vi "Update p PAA25.vi"(8 "error in":errorcluster, 10 "p PAA-25":waveform(dbl)[](array[waveform]), 11 "DeepU Results in":refnum<class "DeepU Results.lvclass">) -> (0 "error out":errorcluster, 3 "DeepU Results out":refnum<class "DeepU Results.lvclass">)   [LabVIEW 2019, in "Results.lvlib" / "DeepU Results.lvclass"]
uses:
  DeepU Results.lvclass
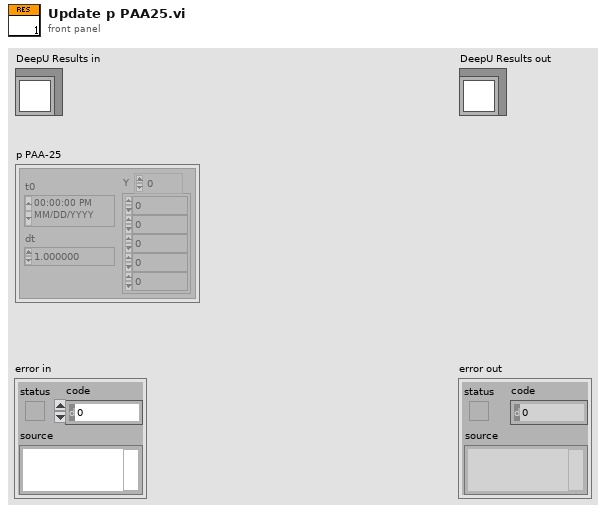
[diagram p1: front panel]
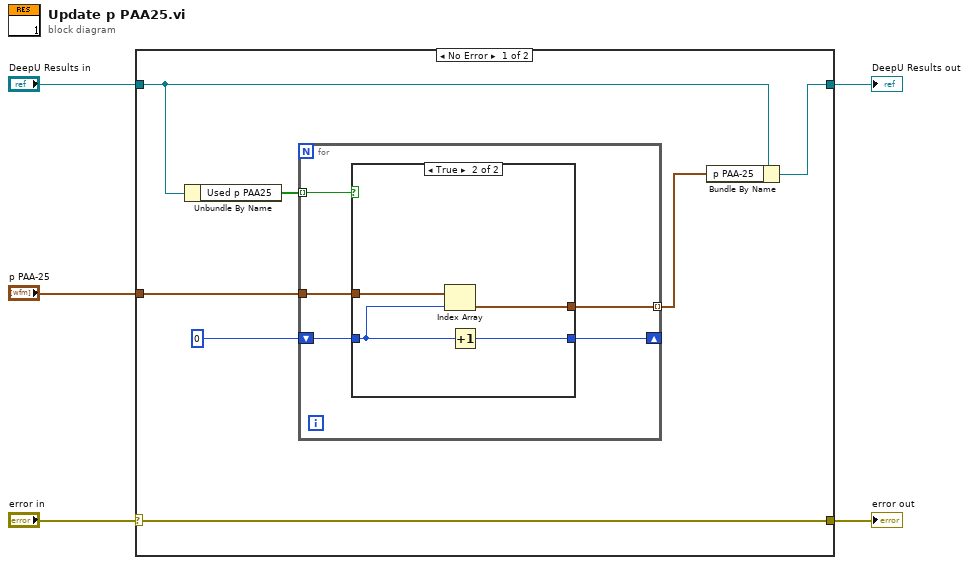
[diagram p0: block diagram]
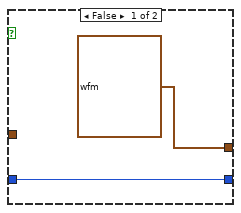
[diagram p2: hidden frame]
diagram:
  n1 = case shown="No Error" "error in" {
    selector: "error in" -> [w12 w24]
    tunnel: [w12 w24] -> w1
    tunnel: [w11 w25] -> w2
    tunnel: "DeepU Results in" -> [w10 w25]
    tunnel: "p PAA-25" -> [w9 _]
    frame No Error {
      n2 = Unbundle By Name(w10) -> ("Used p PAA25"=w6:bool[])
      n3 = for {
        tunnel: w6 -> [w16] mode=indexing
        tunnel: w9 -> [w17]
        shift-right: [w13] -> _
        shift-left: 0 -> [w15]
        tunnel: [w14] -> w7 mode=indexing
        n4 = case shown="True" w16 {
          tunnel: w17 -> [_ w23]
          tunnel: w15 -> [w18 w21]
          tunnel: [waveform(dbl) {"t0"=timestamp(0 s since 1904-01-01), "dt"=1.0, "Y"=[]} ("Waveform") w22] -> w14
          tunnel: [w18 w20] -> w13
          frame False {
          }
          frame True {
            n5 = Index Array(array=w23, index=w21) -> (element=w22:waveform(dbl))
            n6 = Increment(x=w21) -> (x+1=w20:i32)
          }
        }
      }
      n7 = Bundle By Name(cluster=w10, "p PAA-25"=w7) -> (w11:refnum<class "DeepU Results.lvclass">)
    }
    frame Error {
    }
  }
  "error out" <- w1
  "DeepU Results out" <- w2
